vi "Initialize XNET Tree.vi"(8 "error in":errorcluster, 9 "XNET Cluster":refnum<k21>, 10 "XNET Database":refnum<k21>, 11 "Tree":refnum<vi>) -> (0 "error out":errorcluster, 1 "Parent":string, 2 "XNET Cluster Out":refnum<k21>, 3 "Tree Out":refnum<vi>)   [LabVIEW 2019, in "Ghost Bus Addon System Explorer.lvlib"]
uses:
  Ghost Bus Addon System Explorer.lvlib
  <resource>/objmgr/xnet.rc
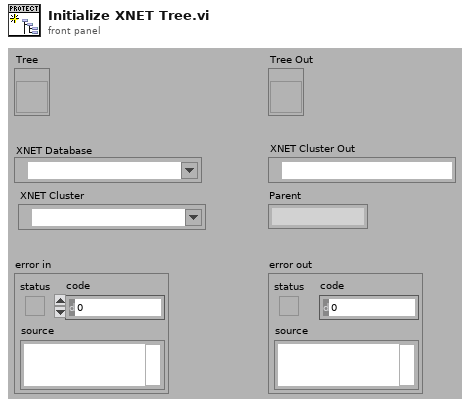
[diagram p1: front panel]
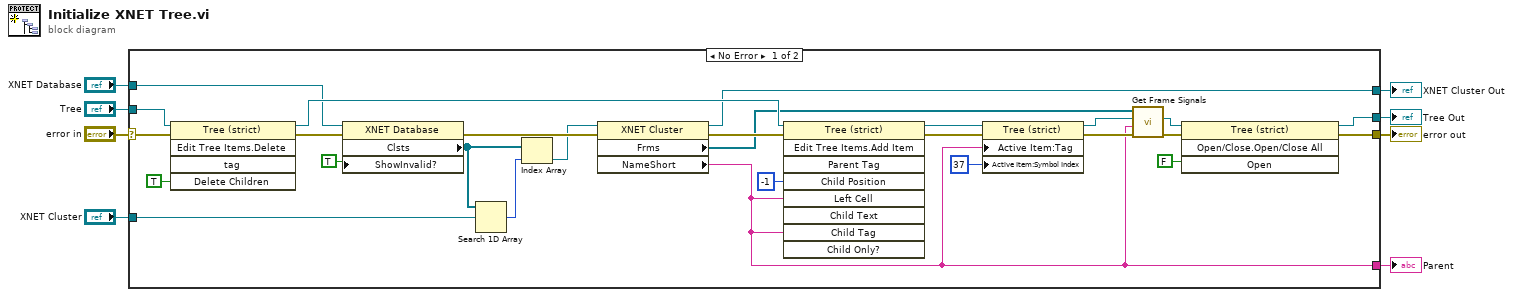
[diagram p0: block diagram]
diagram:
  n1 = case shown="No Error" "error in" {
    selector: "error in" -> [w9 w38]
    tunnel: "Tree" -> [w34 w37]
    tunnel: [w10 w38] -> w7
    tunnel: "XNET Database" -> [w19 _]
    tunnel: [w22 w37] -> w4
    tunnel: [w24 w36] -> w3
    tunnel: "XNET Cluster" -> [w15 w36]
    tunnel: [w11 _] -> w1
    frame No Error {
      n2 = invoke on="Invoke Node" class="Tree (strict)" method="Edit Tree Items.Delete"(reference=w34, error in=w9, "Delete Children"=TRUE ("Delete Children?")) -> (reference out=w35:refnum<vi>, error out=w17:errorcluster)  [unwired: 2 in, 3 out]
      n3 = property class="XNET Database"(reference=w19, error in=w17, "ShowInvalid?"=TRUE ("Show Invalid From Open?")) -> (error out=w16:errorcluster, "Clsts"=w13:refnum<k21>[])  [unwired: 1 out]
      n4 = Search 1D Array(1D array=w13, element=w15) -> (index of element=w14:i32)  [unwired: 1 in]
      n5 = Index Array(array=w13, index=w14) -> (element=w12:refnum<k21>)
      n6 = property class="XNET Cluster"(reference=w12, error in=w16) -> (reference out=w24:refnum<k21>, error out=w26:errorcluster, "Frms"=w25:refnum<k21>[], "NameShort"=w11:string)
      n7 = invoke on="Invoke Node" class="Tree (strict)" method="Edit Tree Items.Add Item"(reference=w35, error in=w26, "Child Position"=-1, "Left Cell"=w11, "Child Tag"=w11) -> (reference out=w29:refnum<vi>, error out=w28:errorcluster)  [unwired: 4 in, 7 out]
      n8 = property class="Tree (strict)"(reference=w29, error in=w28, "Active Item:Tag"=w11, "Active Item:Symbol Index"=37) -> (reference out=w30:refnum<vi>, error out=w31:errorcluster)
      n9 = call "Get Frame Signals.vi"("error in"=w31, "Parent Tag"=w11, "Tree Reference"=w30, "Frms"=w25) -> ("error out"=w21:errorcluster, "Tree Reference Out"=w20:refnum<vi>)  [unwired: 6 in]
      n10 = invoke on="Invoke Node" class="Tree (strict)" method="Open/Close.Open/Close All"(reference=w20, error in=w21, "Open"=FALSE ("Open?")) -> (reference out=w22:refnum<vi>, error out=w10:errorcluster)  [unwired: 1 in, 2 out]
    }
    frame Error {
    }
  }
  "error out" <- w7
  "Tree Out" <- w4
  "XNET Cluster Out" <- w3
  "Parent" <- w1
